vi "LS4 SetVelSingleAxis_SD.vi"(1 "Vel":dbl format="%.2f", 2 "Axis":i32=1) -> (0 "Command executed":bool)   [LabVIEW 2015]
uses:
  DLL/LStep4.dll
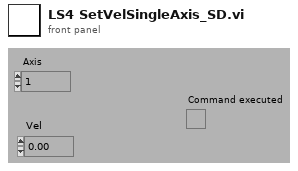
[diagram p1: front panel]
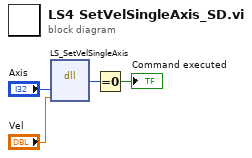
[diagram p0: block diagram]
diagram:
  n1 = dll-call lib="G:/SD/TRANCON-2015/DLL/LStep4.dll" fn="LS_SetVelSingleAxis"("Axis"="Axis", "Vel"="Vel") -> ("type de retour"=w3:i32)  [unwired: 5 in, 2 out]
  n2 = Equal To 0?(x=w3) -> (x = 0?=→"Command executed":bool)
